vi "Read_Image(Batch).vi"(5 "mBatch":i32, 6 "PreProcessing_Options":T1={"DS_Name"="", "Input_Dims"={"C"=0, "H"=224, "W"=224}, "Center Crop Size"=-1, "Interpolation Type"=1, "Dataset_Stats"={"means"={"R"=0.5385, "G"=0.5348, "B"=0.551}, "stds"={"R"=0.3673, "G"=0.3673, "B"=0.3505}}} {"Dataset_Stats"."stds"."R" format="%#_3g"; "Dataset_Stats"."stds"."G" format="%#_3g"; "Dataset_Stats"."stds"."B" format="%#_3g"; "Dataset_Stats"."means"."R" format="%#_3g"; "Dataset_Stats"."means"."G" format="%#_3g"; "Dataset_Stats"."means"."B" format="%#_3g"; "Interpolation Type" items=["Zero Order", "Bi-Linear", "Quadratic", "Cubic Spline"]}, 7 "Dataset_Stats":T3[](array[typedef]) {"stds"."R" format="%#_3g"; "stds"."G" format="%#_3g"; "stds"."B" format="%#_3g"; "means"."R" format="%#_3g"; "means"."G" format="%#_3g"; "means"."B" format="%#_3g"}, 8 "error in":errorcluster, 9 "index":i32, 10 "Dims_In":T2, 11 "Array":path[][](array[path])) -> (0 "error out":errorcluster, 2 "dT_Img_Read":dbl format="%0.2f", 3 "Image(Batch) Out":sgl[][][][](array[numeric]))   [LabVIEW 2024]
uses:
  <vilib>/Analysis/NI_AALBase.lvlib
  <vilib>/Analysis/baseanly.llb/Mean (DBL).vi
  DeepLTK_Anomaly_Detection_Addon/API/Controls/Image_Stats_RGB.ctl
  DeepLTK_Anomaly_Detection_Addon/API/Controls/NNPC_DS_Stats.ctl
  <vilib>/Ngene/Deep Learning Toolkit/Toolkit/NN_Data/API/NN_Dims(C,H,W).ctl
  <vilib>/Ngene/Deep Learning Toolkit/Toolkit/Deep_Learning_Toolkit_by_Ngene.lvlib
  DeepLTK_Anomaly_Detection_Addon/API/Controls/NNPC_PreProcessing_Options.ctl
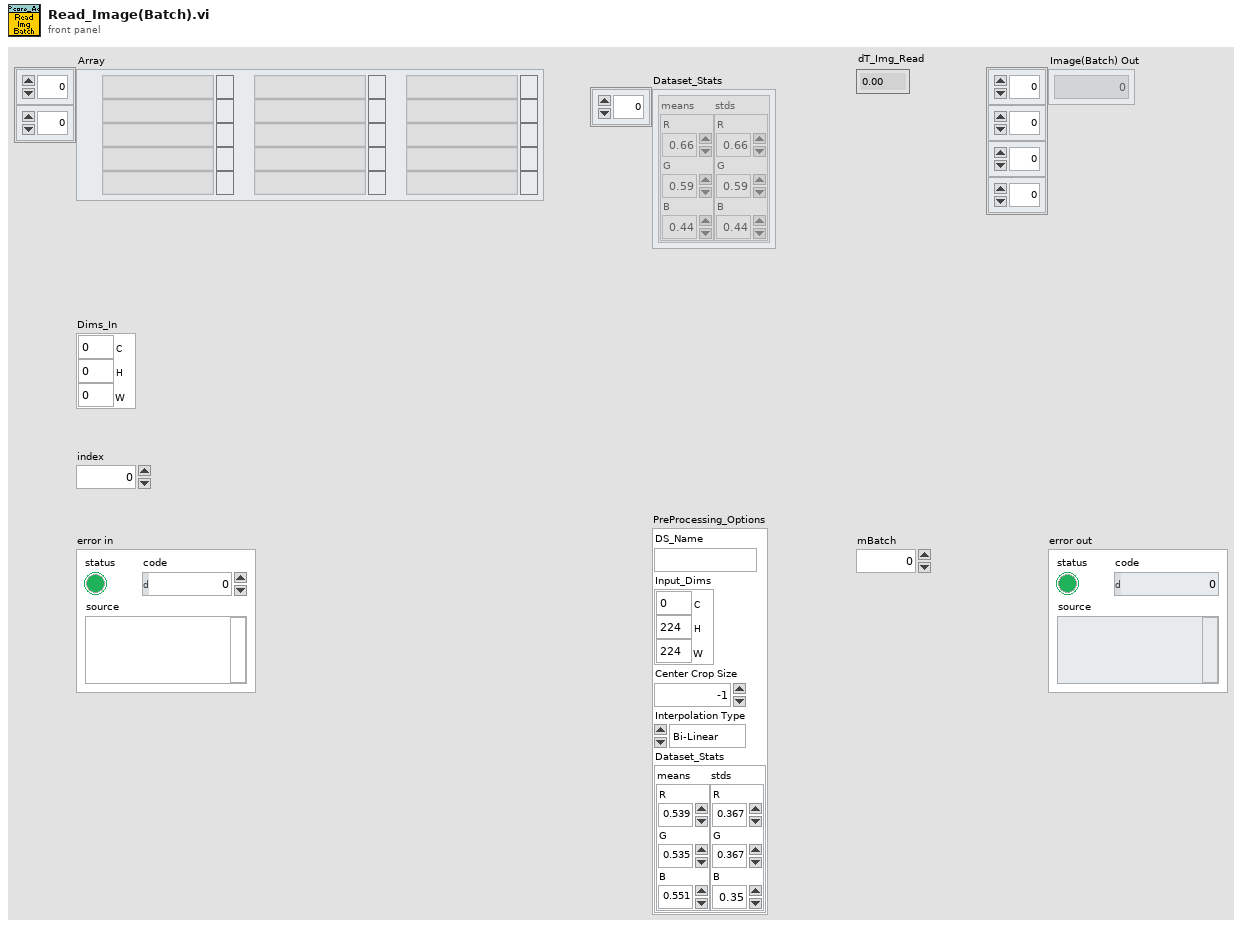
[diagram p1: front panel]
types:
  T1 = typedef "NNPC_PreProcessing_Options.ctl" = cluster{"DS_Name":string, "Input_Dims":T2, "Center Crop Size":i32, "Interpolation Type":u32, "Dataset_Stats":T3}
  T2 = typedef "Deep_Learning_Toolkit_by_Ngene.lvlib/NN_Dims(C,H,W).ctl" = cluster{"C":i32, "H":i32, "W":i32}
  T3 = typedef "NNPC_DS_Stats.ctl" = cluster{"means":T4, "stds":T4}
  T4 = typedef "Image_Stats_RGB.ctl" = cluster{"R":sgl, "G":sgl, "B":sgl}
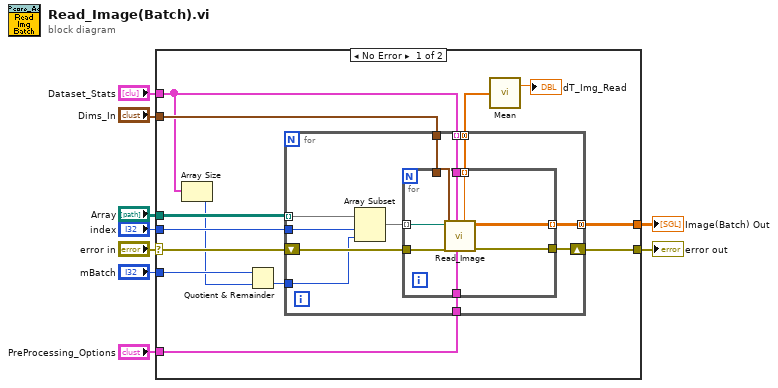
[diagram p0: block diagram]
diagram:
  n1 = case shown="No Error" "error in" {
    selector: "error in" -> [w14 w42]
    tunnel: [w22 _] -> w9
    tunnel: [w21 w42] -> w8
    tunnel: "Dataset_Stats" -> [w12 _]
    tunnel: "Dims_In" -> [w20 _]
    tunnel: "Array" -> [w19 _]
    tunnel: "PreProcessing_Options" -> [w18 _]
    tunnel: "index" -> [w17 _]
    tunnel: "mBatch" -> [w13 _]
    frame No Error {
      n2 = Array Size(array=w12) -> (size(s)=w11:i32)
      n3 = Quotient & Remainder(x=w13, y=w11) -> (floor(x/y)=w10:i32)  [unwired: 1 out]
      n4 = for {
        tunnel: [w32] -> w16 mode=concatenating
        tunnel: w19 -> [w25] mode=indexing
        tunnel: [w31] -> w22 mode=concatenating
        tunnel: w12 -> [w29] mode=indexing
        tunnel: w20 -> [w28]
        tunnel: w18 -> [w27]
        shift-right: [w30] -> w21
        shift-left: w14 -> [w33]
        tunnel: w17 -> [w24]
        tunnel: w10 -> [w23]
        n5 = Array Subset(array=w25, index=w24, length=w23) -> (w26:path[])
        n6 = for {
          tunnel: w33 -> [w41]
          tunnel: [w40] -> w32 mode=indexing
          tunnel: w26 -> [w39] mode=indexing
          tunnel: [w38] -> w31 mode=indexing
          tunnel: [w37] -> w30
          tunnel: w29 -> [w36]
          tunnel: w28 -> [w35]
          tunnel: w27 -> [w34]
          n7 = call "Read_Image.vi"(6:w34, "PreProcessing_Options"=w36, "error in"=w41, "IMAQ Name"=w35, "Img Path"=w39) -> ("error out"=w37:errorcluster, "Image Out"=w38:sgl[][][], "dT_Img_Read"=w40:dbl)  [unwired: 3 in, 1 out]
        }
      }
      n8 = call-poly <vilib>:"Mean.vi"("X"=w16) -> ("mean"=→"dT_Img_Read":dbl)  [unwired: 1 out]
    }
    frame Error {
    }
  }
  "Image(Batch) Out" <- w9
  "error out" <- w8
